vi "WILT Update Wilt GUI.vi"(0 "Dryer In":T1 {"Night Cycle Count" format="%04d"; "Day Cycle Count" format="%04d"}, 1 "Day Shift?":bool, 2 "Enum":T7, 3 "Station Index":i32=13, 5 "Station Label In":string, 7 "New Dryer Details In":T2, 9 "Com Port In":u8=13, 11 "Dryer Status Serial Data In":T5, 12 "Agilent Data In":dbl[](array[numeric])=[1.0, 2.0, 3.0, 4.0, 5.0], 13 "Audit Alert":bool) -> (4 "Dryer Out 2":T1 {"Night Cycle Count" format="%04d"; "Day Cycle Count" format="%04d"}, 8 "New Dryer Testing File Init":bool, 10 "Restart Ready?":bool)   [LabVIEW 2016]
uses:
  Type Definitions/WILT Dryer Status Ctrl.ctl
  Globals/Globals Wilt.vi
  Type Definitions/WILT Dryer.ctl
  Type Definitions/WILT Dryer Details.ctl
  Type Definitions/WILT Dryer Com Port Info.ctl
  Type Definitions/WILT Update GUI Control.ctl
  Type Definitions/WILT Agilent Channel Definition.ctl
  Type Definitions/WILT DAQ Data.ctl
panel:
  in  "Tab Control":enum32{"Out", "In"}(tab)
  out "Dryer Breakout":T1 {"Night Cycle Count" format="%04d"; "Day Cycle Count" format="%04d"}
  in  "Dryer Out":T1 {"Night Cycle Count" format="%04d"; "Day Cycle Count" format="%04d"}
  out "Dryer Breakout":T1 {"Night Cycle Count" format="%04d"; "Day Cycle Count" format="%04d"}
  in  "Dryer":T1 {"Night Cycle Count" format="%04d"; "Day Cycle Count" format="%04d"}
  # "Day"
  # "Night"
  # "Day"
  # "Night"
  # "Day"
  # "Night"
  # "Day"
  # "Night"
  # "Day"
  # "Night"
  # "Day"
  # "Night"
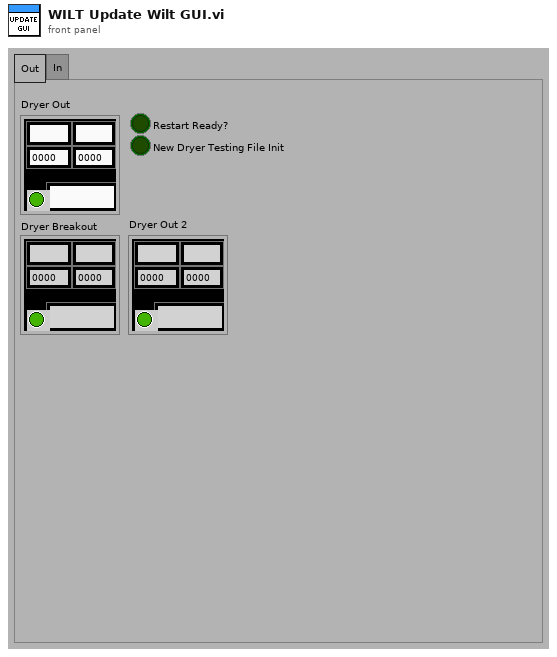
[diagram p1: front panel]
types:
  T1 = typedef "WILT Dryer.ctl" = cluster{"Lab ID":string, "Day Cycle Count":i32, "Station Label":string, "Dryer Details":T2, "Status Color":u32, "Invisible Button":bool, "Night Cycle Count":i32, "Station Index":i32, "Cycle Index":string, "Audit Alert":bool, "Agilent Channel Definition":T3, "DAQ Data":T4}
  T2 = typedef "WILT Dryer Details.ctl" = cluster{"Station":string, "Lab ID":string, "TR Number":string}
  T3 = typedef "WILT Agilent Channel Definition.ctl" = cluster{"Channel":string, "Station":string, "Label":string, "Agilent Station":string, "Data":dbl}
  T4 = typedef "WILT DAQ Data.ctl" = cluster{"L1 Current":dbl, "L2 Current":dbl, "Temperature  Deg F (TC)":dbl, "Volts":dbl, "Volts (208)":dbl, "SW (208)":dbl}
  T5 = typedef "WILT Dryer Com Port Info.ctl" = cluster{"Color":u32, "Last Read Status":T6, "Command:Data":string, "Com Port":u8, "Time(S)":dbl, "Err Count":u32}
  T6 = typedef "WILT Dryer Status Ctrl.ctl" = enum16{"Cycle Not Started", "Cycle Running", "Paused", "Cycle Completed", "Eval Mode Entered", "Err", "Pause (No GEA2)"}
  T7 = typedef "WILT Update GUI Control.ctl" = enum16{"Init Station Number", "Update Detail Data", "Update Status", "Init Com Port Num", "Update Sample Info", "Reset All Cycles"}
  T8 = cluster{"New Dryer Details In":T2, "Station Label In":string, "Com Port In":u8, "Agilent Data In":dbl[], "Dryer Status Serial Data In":T5, "Restart Ready?":bool, "Dryer Out":T1, "Temperature Fault":bool, "Station Index":i32, "Audit Alert":bool, "Day Shift?":bool}
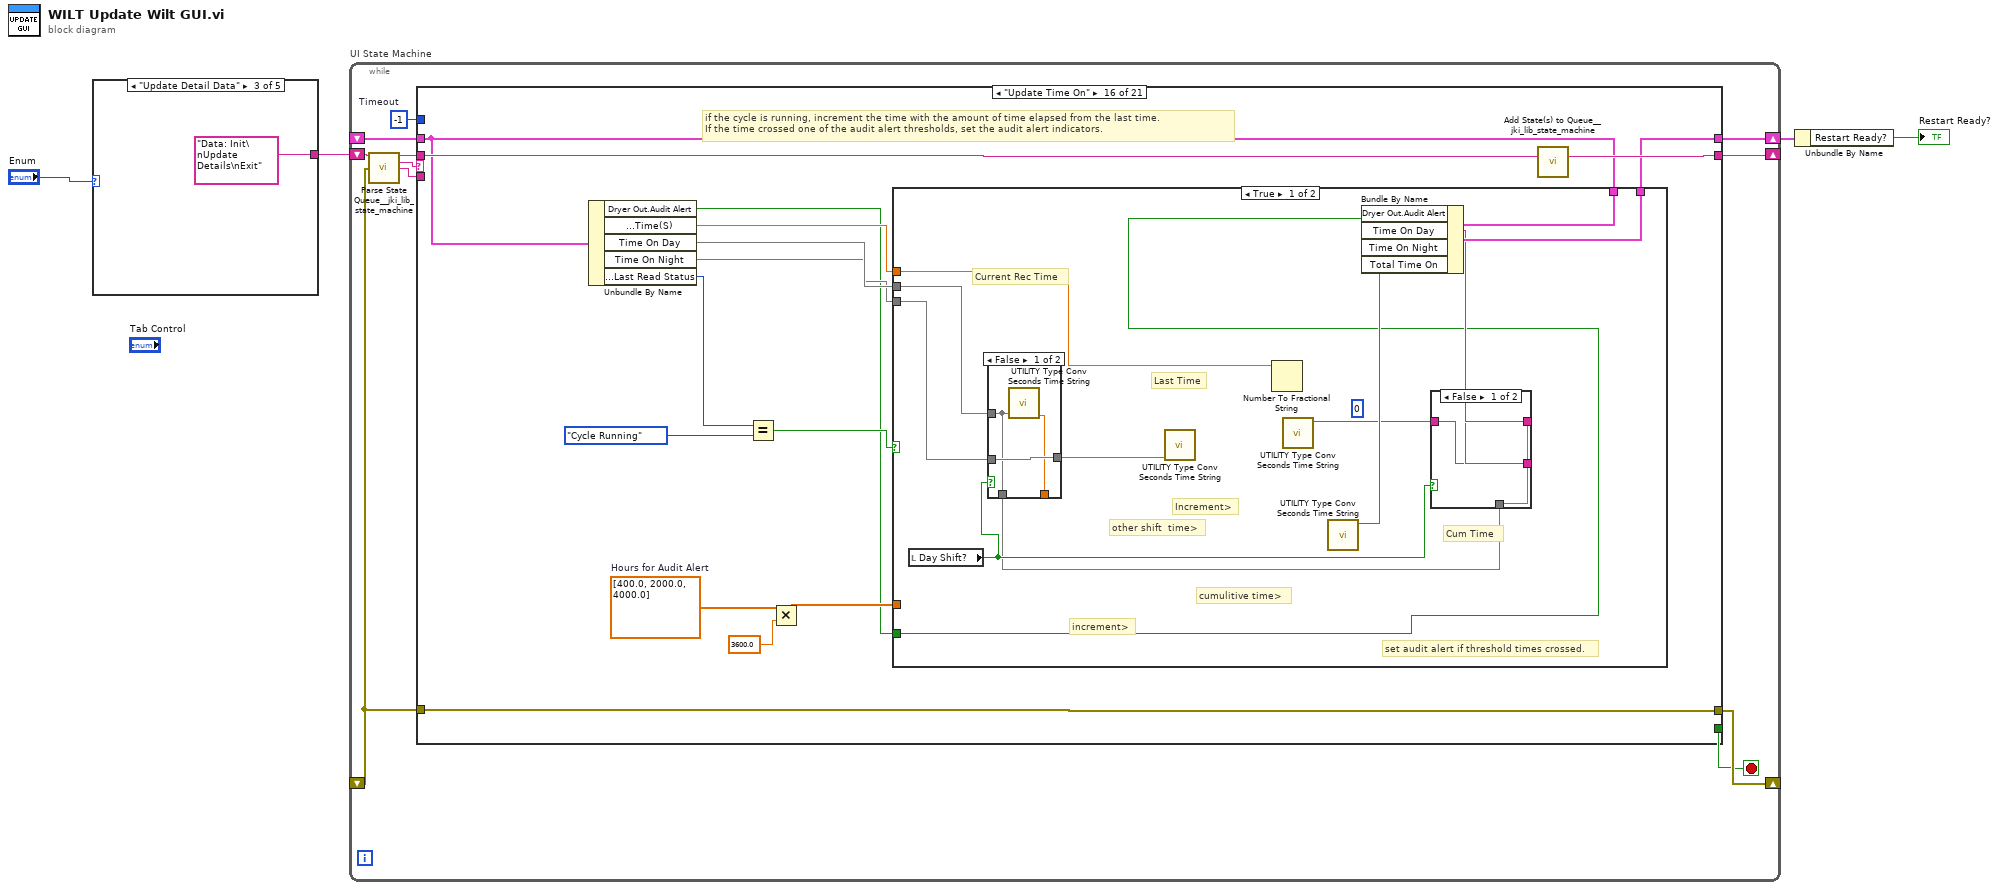
[diagram p0: block diagram]
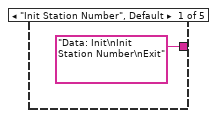
[diagram p2: hidden frame]
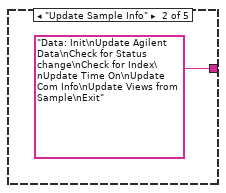
[diagram p3: hidden frame]
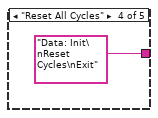
[diagram p4: hidden frame]
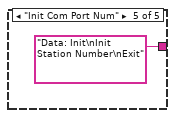
[diagram p5: hidden frame]
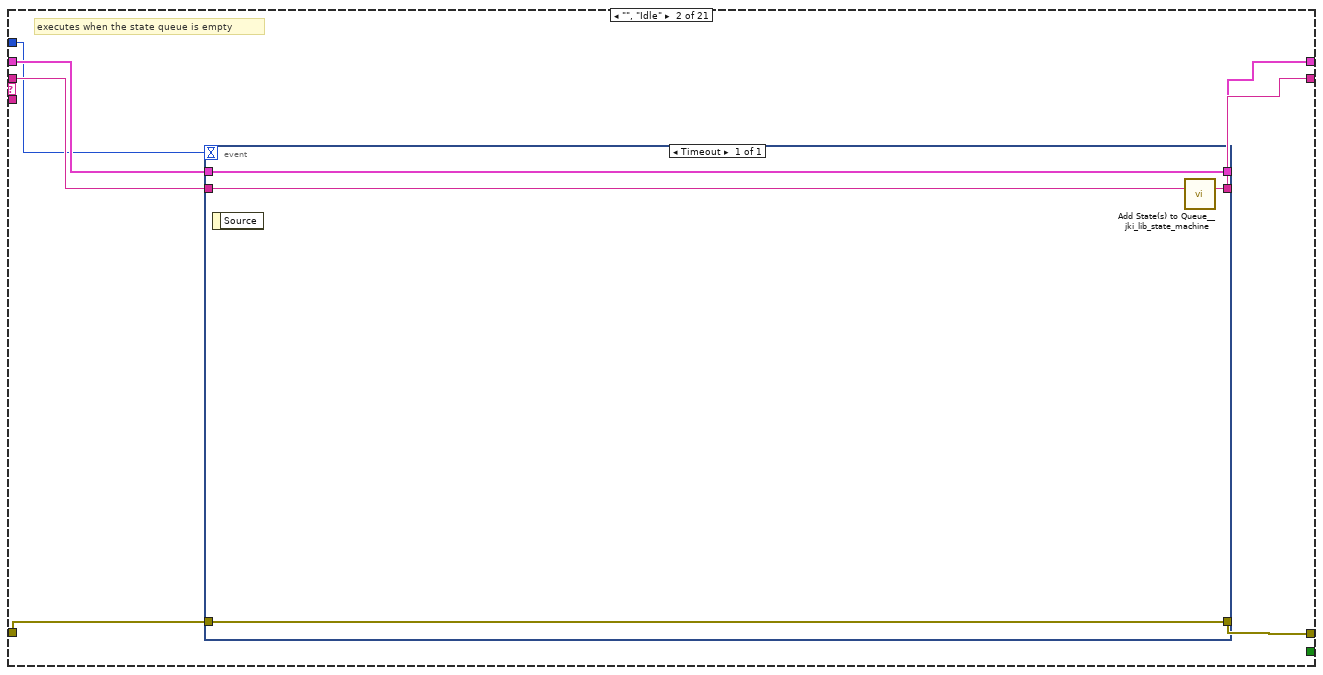
[diagram p7: hidden frame]
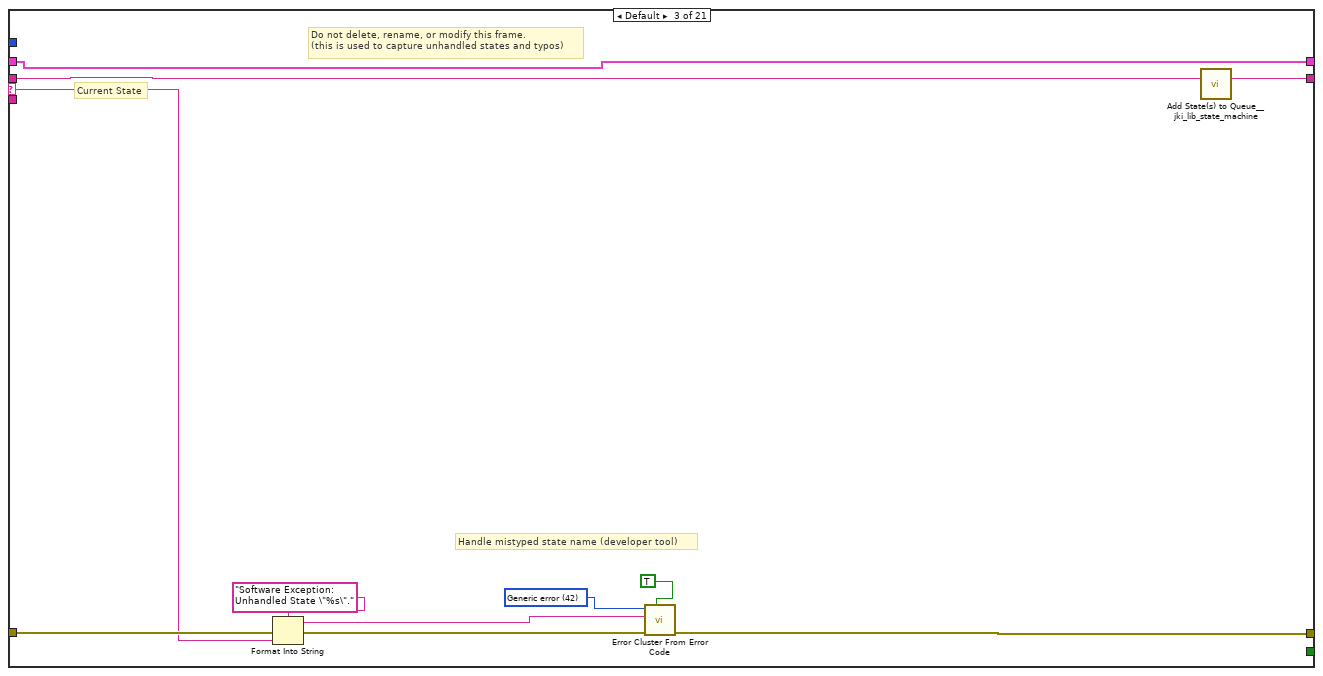
[diagram p8: hidden frame]
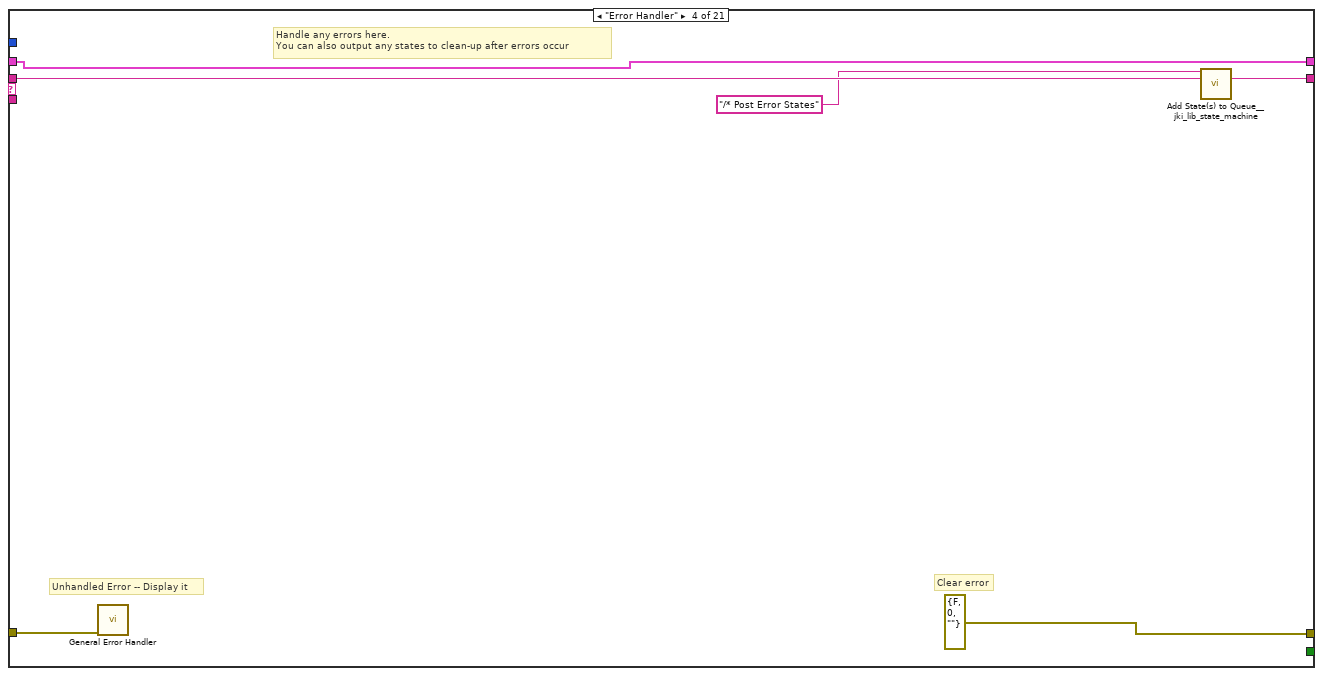
[diagram p9: hidden frame]
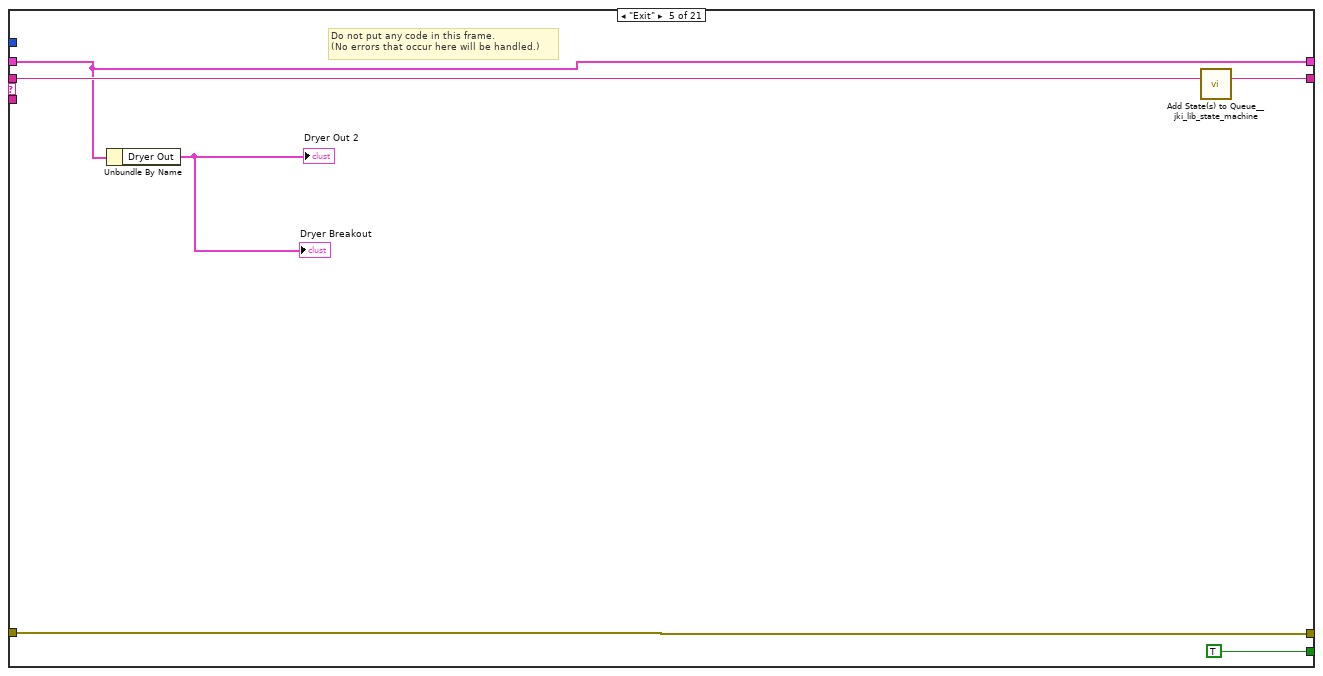
[diagram p10: hidden frame]
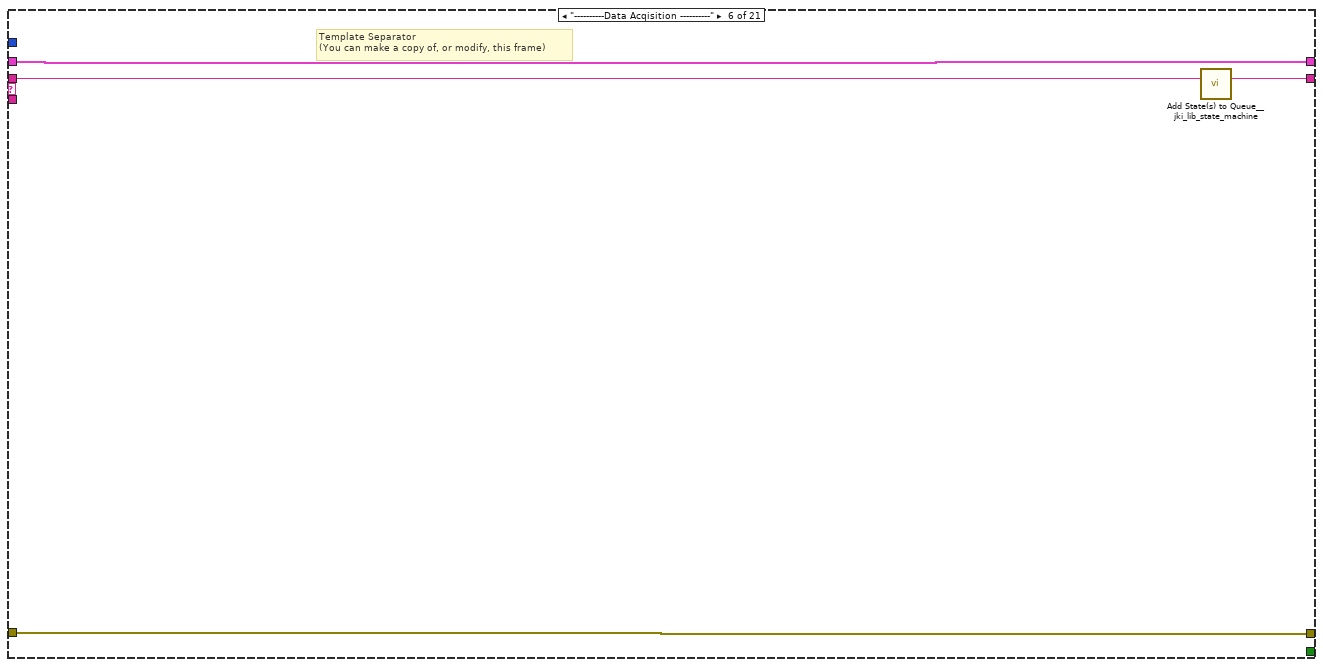
[diagram p11: hidden frame]
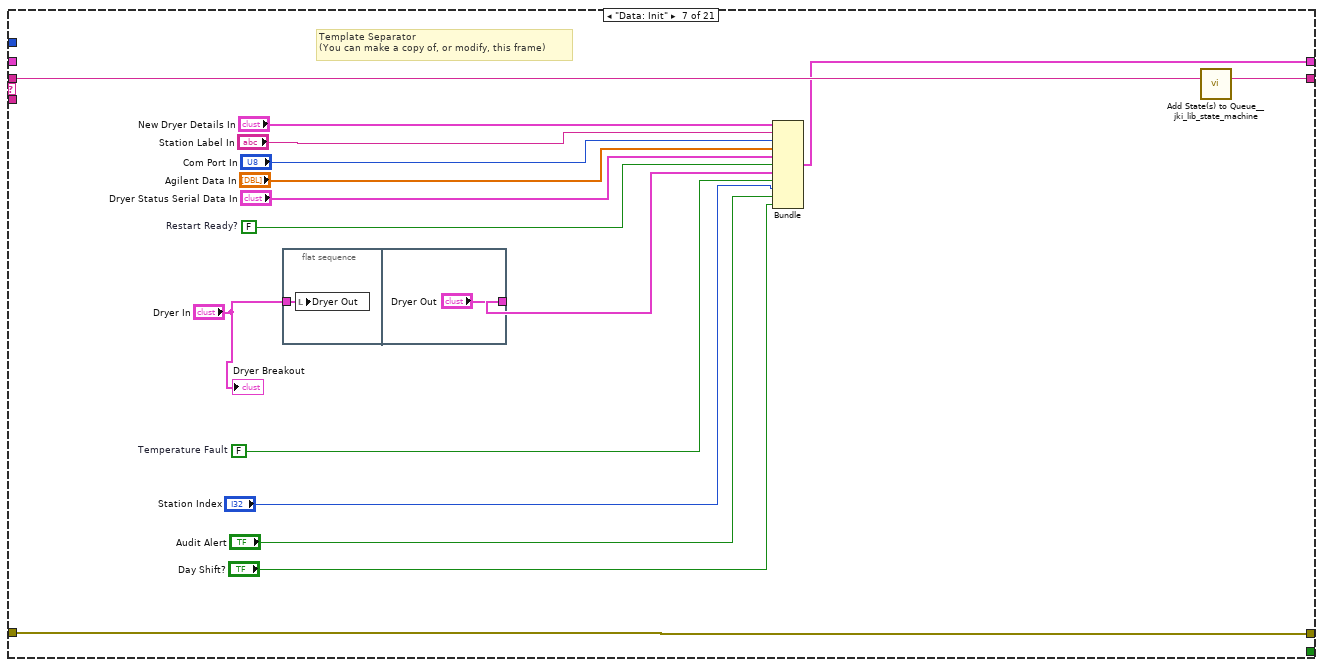
[diagram p12: hidden frame]
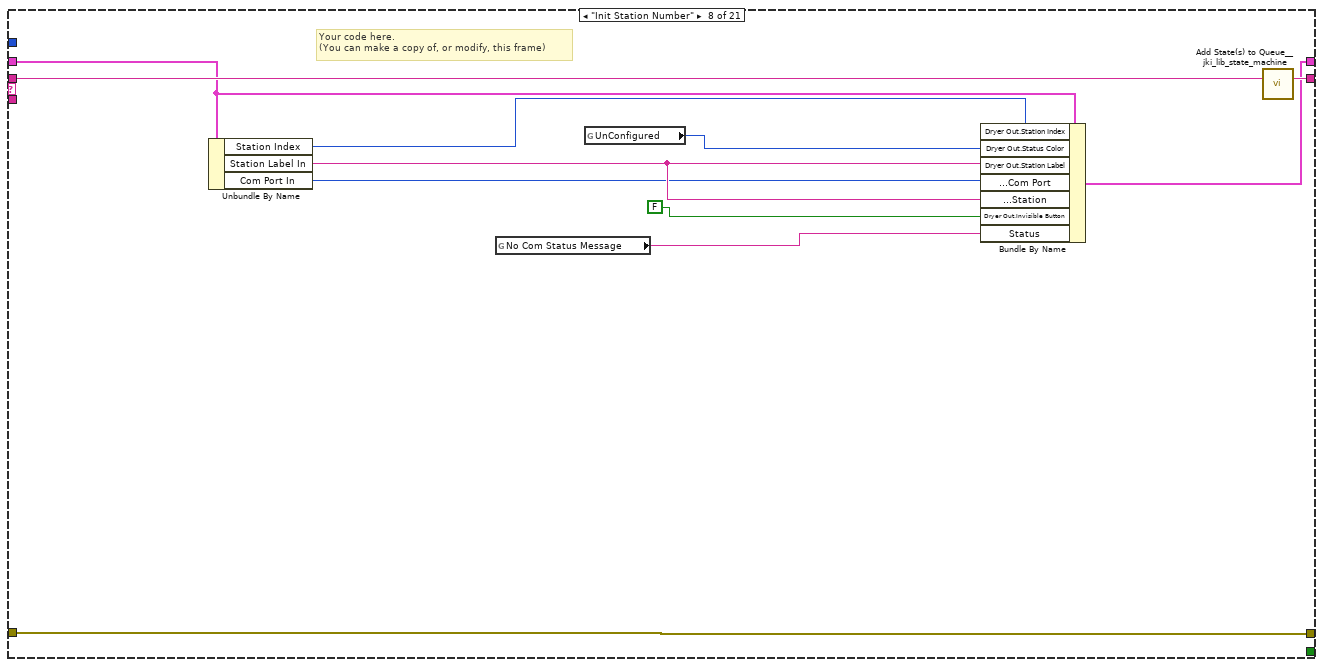
[diagram p13: hidden frame]
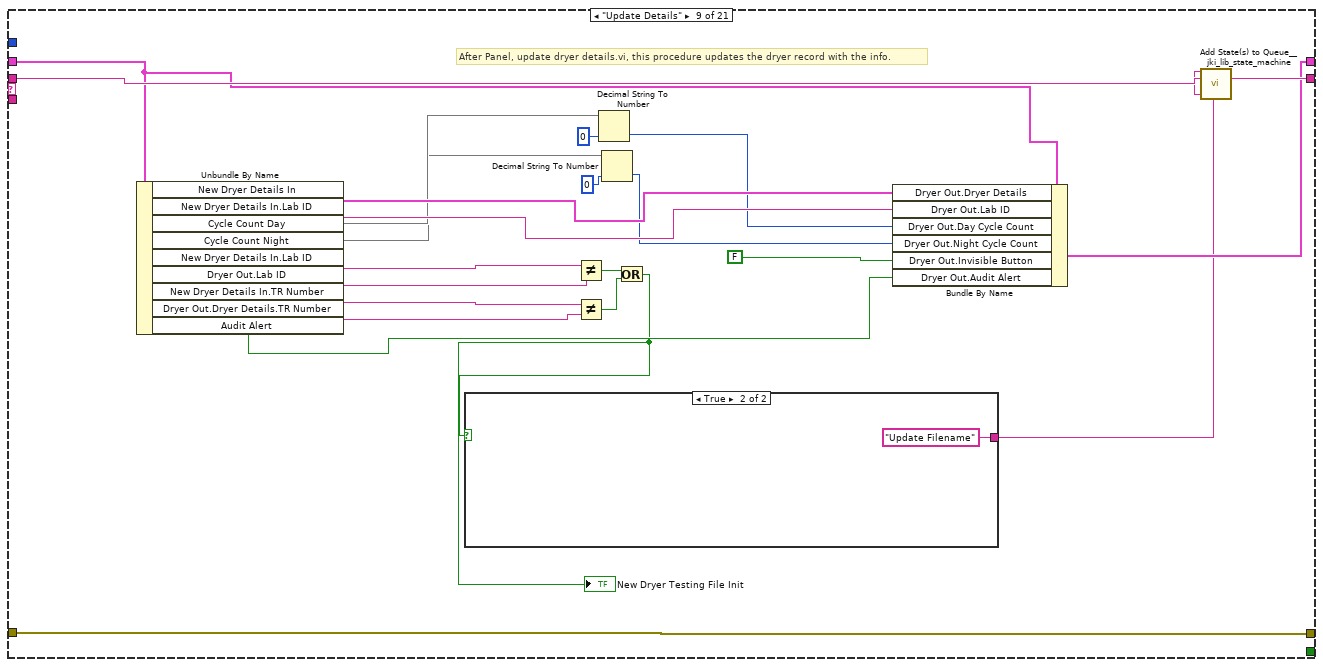
[diagram p14: hidden frame]
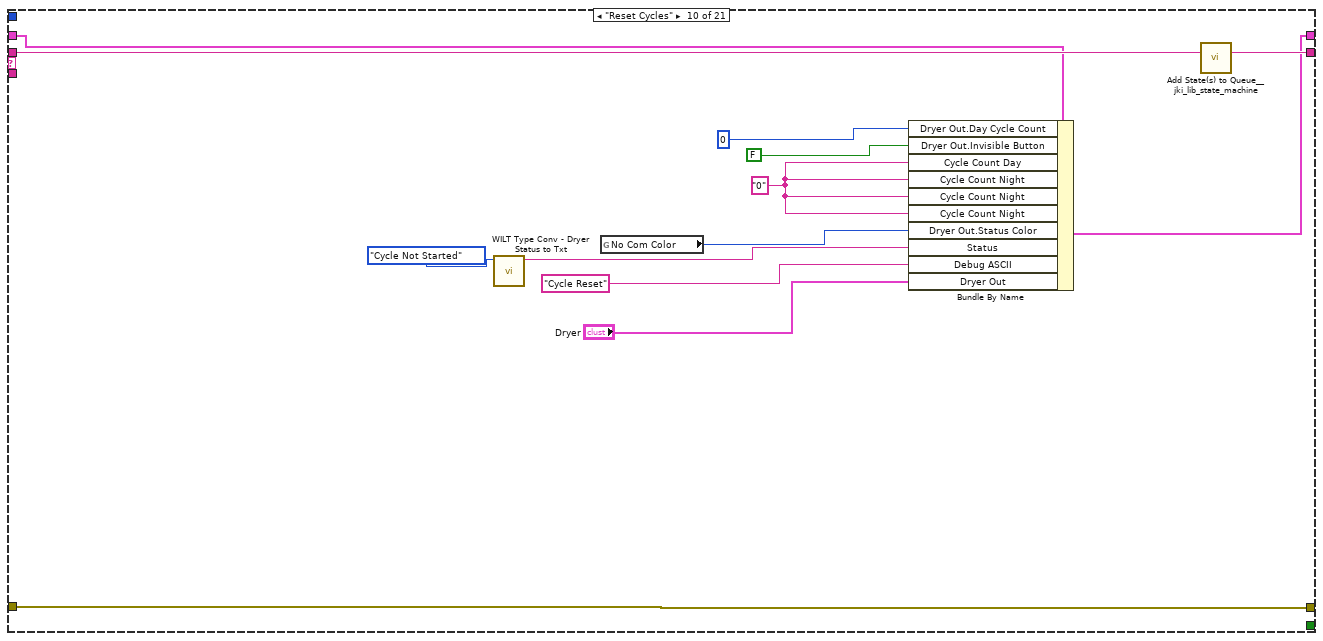
[diagram p16: hidden frame]
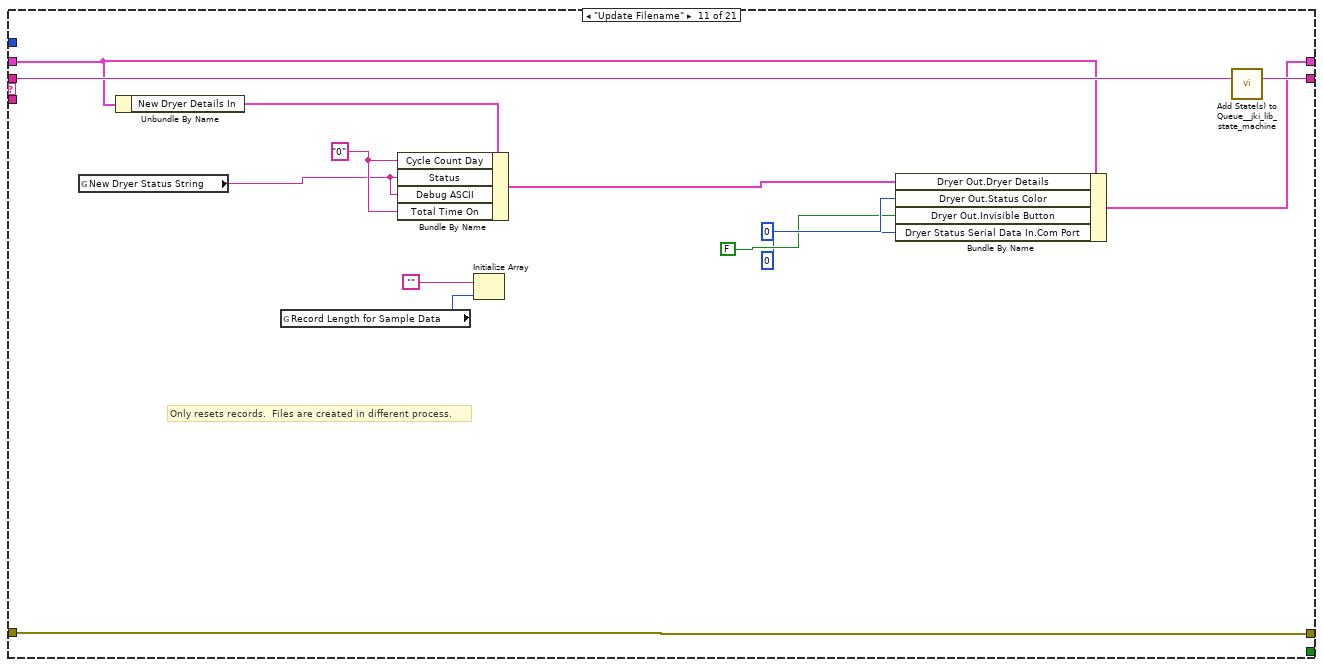
[diagram p17: hidden frame]
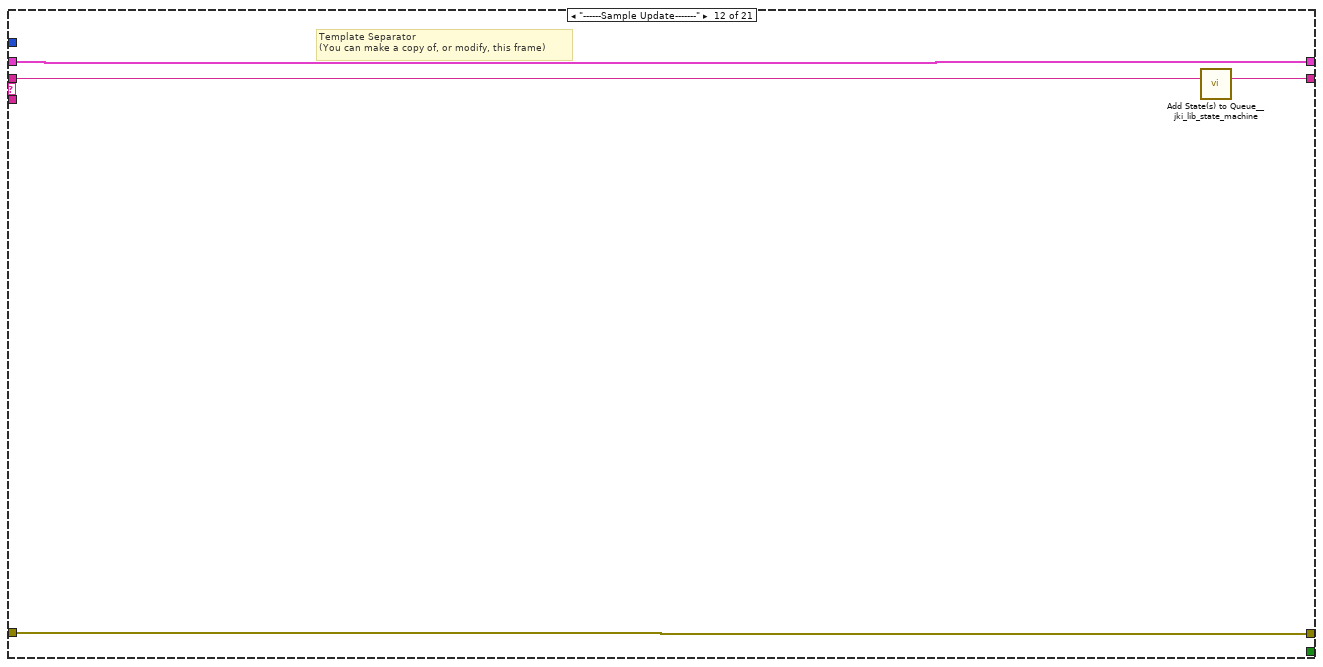
[diagram p18: hidden frame]
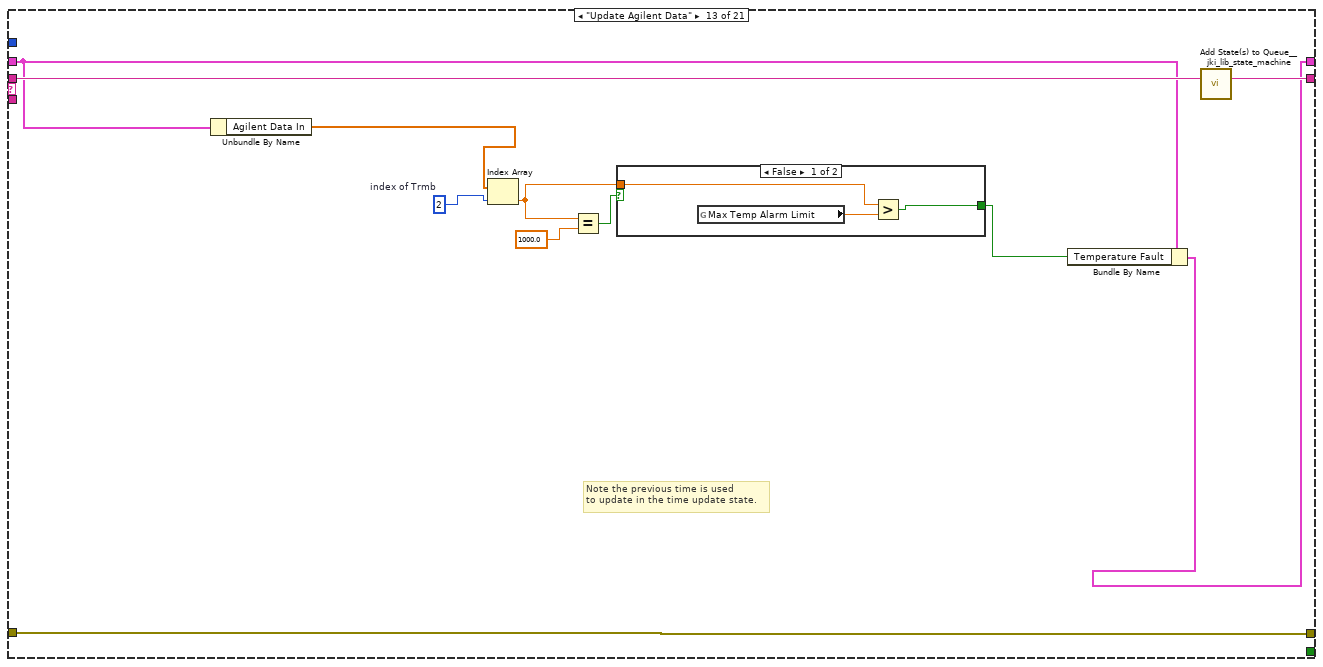
[diagram p19: hidden frame]
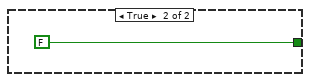
[diagram p20: hidden frame]
diagram:
  n1 = case shown="\"Update Detail Data\"" "Enum" {
    tunnel: ["Data: Init\nInit Station Number\nExit" ("States Out") "Data: Init\nUpdate Agilent Data\nCheck for Status change\nCheck for Index\nUpdate Time On\nUpdate Com Info\nUpdate Views from Sample\nExit" ("States Out") "Data: Init\nUpdate Details\nExit" ("States Out") "Data: Init\nReset Cycles\nExit" ("States Out") "Data: Init\nInit Station Number\nExit" ("States Out")] -> w3
    frame "Init Station Number", Default {
    }
    frame "Update Sample Info" {
    }
    frame "Update Detail Data" {
    }
    frame "Reset All Cycles" {
    }
    frame "Init Com Port Num" {
    }
  }
  n2 = while "UI State Machine" {
    shift-right: [w13] -> w2
    shift-left: _ -> [w12]
    shift-right: [w16] -> _
    shift-left: _ -> [w10]
    shift-right: [w15] -> _
    shift-left: w3 -> [w17]
    stop <- w14 stop-if-true
    w11 = -1  # Timeout
    n3 = call <vilib>:"Parse State Queue__jki_lib_state_machine.vi"("State Queue"=w17, "Error In (no error)"=w10) -> ("Remaining States"=w19:string, "Current State"=w20:string, "Arguments"=w18:string)  [unwired: 11 in]
    n4 = case shown="\"Update Time On\"" w20 {
      selector: w20 -> [_ _ w35 _ _ _ _ _ _ _ _ _ _ _ _ _ _ _ _ _ _]
      tunnel: w19 -> [w22 w30 w39 w51 w57 w61 w77 w90 w113 w127 w141 w145 w156 w164 w168 w183 w223 w227 w231 w238 w254]
      tunnel: w18 -> [_ _ _ _ _ _ _ _ _ _ _ _ _ _ _ _ _ _ _ _ _]
      tunnel: w12 -> [w23 w28 w37 w48 w53 w58 _ w80 w106 w117 w138 w142 w152 w161 w165 w178 w220 w224 w228 w232 w251]
      tunnel: [w21 w27 w41 errorcluster {"status"=FALSE, "code"=0, "source"=""} ("error out") w55 w59 w75 w88 w111 w125 w139 w143 w154 w162 w166 w181 w221 w225 w229 w236 w252] -> w16
      tunnel: w10 -> [w21 w26 w40 w47 w55 w59 w75 w88 w111 w125 w139 w143 w154 w162 w166 w181 w221 w225 w229 w236 w252]
      tunnel: [w22 w29 w38 w50 w56 w60 w76 w89 w112 w126 w140 w144 w155 w163 w167 w182 w222 w226 w230 w237 w253] -> w15
      tunnel: [_ _ _ _ TRUE _ _ _ _ _ _ _ _ _ _ _ _ _ _ _ _] -> w14
      tunnel: [w23 w25 w37 w48 w53 w58 w74 w87 w110 w124 w137 w142 w146 w161 w165 w177 w219 w224 w228 w232 w250] -> w13
      tunnel: w11 -> [_ w24 _ _ _ _ _ _ _ _ _ _ _ _ _ _ _ _ _ _ _]
      frame "ABOUT" {
        # "TAKES DATA FROM DRYER COM INFO AND INTEGRATES IT INTO THE RECORD."
        # "Update Dryer WILT data structure\nwith new data, or init:"
      }
      frame "", "Idle" {
        # "executes when the state queue is empty"
        n5 = event shown="[0] Timeout" {
          selector: _ -> [_]
          dyn-events: _ -> [_]
          timeout: w24 -> [_]
          tunnel: w30 -> [w34]
          tunnel: [w33] -> w29
          tunnel: w28 -> [w31]
          tunnel: [w32] -> w27
          tunnel: w26 -> [w32]
          tunnel: [w31] -> w25
          event Timeout {
            n6 = event-data() -> ()  [unwired: 1 in, 1 out]
            n7 = call <vilib>:"Add State(s) to Queue__jki_lib_state_machine.vi"("State(s) in (\"\")"=w34) -> ("States Out"=w33:string)  [unwired: 14 in]
          }
        }
      }
      frame Default {
        w44 = 42 items=["No error", "Argument error", "Memory is full", "Out of zone", "End of file", "File already open", "Generic file I/O error", "File not found", "File permission error", "Disk is full", "Duplicate path", "Too many files open", "System feature not enabled", "Resource file not found", "Cannot add resource", "Resource not found", "Image not found", "Image memory error", "Pen does not exist", "Config type invalid", "Config token not found", "Config parse error", "Config memory error", "Bad external code format", "Bad external code offset", "External code not present", "Null window", "Destroy window error", "Null menu", "Print aborted", "Bad print record", "Print driver error", "Windows error during printing", "Memory error during printing", "Print dialog error", "Generic print error", "Invalid device refnum", "Device not found", "Device parameter error", "Device unit error", "Cannot open device", "Device call aborted", "Generic error", "Cancelled by user", "Object ID too low", "Object ID too high", "Object not in heap", "Unknown heap", "Unknown object (invalid DefProc)", "Unknown object (DefProc not in table)", "Message out of range", "Invalid (null) method", "Unknown message", "Manager call not supported", "Bad address", "Network operation in progress", "Network operation timed out", "Connection is busy", "Network attribute not supported", "Network error", "Address in use", "System out of memory", "Connection aborted", "Connection refused", "Not connected", "Already connected", "Connection closed", "Initialization error (interapplication manager)", "Bad occurrence", "Wait on unbound occurrence handler", "Occurrence queue overflow", "Datalog type conflict", "Unused", "Unrecognized type (interapplication manager)", "Memory corrupt", "Failed to make temporary DLL", "Old CIN version", "Drag socket not found", "Failed to load drop-object", "Failed to register OLE object", "Failed to release OLE object", "Format specifier type mismatch", "Unknown format specifier", "Too few format specifiers", "Too many format specifiers", "Scan failed", "Newer CIN version", "Error converting to variant", "Runtime menu error", "Password tampered", "Variant attribute not found", "Incompatible variant data type", "Event data is not available", "Event Store is not present", "Occurrence is not found", "Event Queue is not created", "Event info is not available", "Refnum passed is NULL", "Error retrieving Class GUID", "Error retrieving CoClass GUID", "Error retrieving TypeLib GUID.", "Bad built application magic bytes.", "Specific driver is different from the specific driver associated with the Logical Name.", "There is no session opened to the class driver.", "Max Error", "MAX - Error with config objects", "MAX - Error loading configuration", "MAX - Group not supported"]
        # "Current State"
        # "Do not delete, rename, or modify this frame.\n(this is used to capture unhandled states and typos)"
        # "Handle mistyped state name (developer tool)"
        n8 = Format Into String(format string="Software Exception: Unhandled State \"%s\"." ("message"), error in=w40, w35) -> (resulting string=w43:string, error out=w42:errorcluster)  [unwired: 1 in]
        n9 = call <vilib>:"Error Cluster From Error Code.vi"("show call chain? (False)"=TRUE, "error in (no error)"=w42, "error message (\"\")"=w43, "error code (0)"=w44) -> ("error out"=w41:errorcluster)  [unwired: 5 in]
        n10 = call <vilib>:"Add State(s) to Queue__jki_lib_state_machine.vi"("State(s) in (\"\")"=w39) -> ("States Out"=w38:string)  [unwired: 14 in]
      }
      frame "Error Handler" {
        # "Unhandled Error -- Display it"
        # "Handle any errors here.\nYou can also output any states to clean-up after errors occur"
        # "Clear error"
        n11 = call <vilib>:"General Error Handler.vi"("error in (no error)"=w47) -> ()  [unwired: 10 in, 5 out]
        n12 = call <vilib>:"Add State(s) to Queue__jki_lib_state_machine.vi"("State(s) in Front (\"\")"="/* Post Error States", "State(s) in (\"\")"=w51) -> ("States Out"=w50:string)  [unwired: 13 in]
      }
      frame "Exit" {
        # "Do not put any code in this frame.\n(No errors that occur here will be handled.)"
        n13 = Unbundle By Name(w53) -> ("Dryer Out"=→"Dryer Out 2" →"Dryer Breakout":T1)
        n14 = call <vilib>:"Add State(s) to Queue__jki_lib_state_machine.vi"("State(s) in (\"\")"=w57) -> ("States Out"=w56:string)  [unwired: 14 in]
      }
      frame "----------Data Acqisition ----------" {
        # "Template Separator\n(You can make a copy of, or modify, this frame)"
        n15 = call <vilib>:"Add State(s) to Queue__jki_lib_state_machine.vi"("State(s) in (\"\")"=w61) -> ("States Out"=w60:string)  [unwired: 14 in]
      }
      frame "Data: Init" {
        w66 = FALSE  # Temperature Fault
        w69 = FALSE  # Restart Ready?
        # "Template Separator\n(You can make a copy of, or modify, this frame)"
        n16 = flat-sequence {
          tunnel: "Dryer In" -> [w78]
          tunnel: ["Dryer Out"] -> w67
          frame #0 {
            n17 = local write "Dryer Out"(w78) -> ()
          }
          frame #1 {
          }
        }
        n18 = Bundle("New Dryer Details In"="New Dryer Details In", "Station Label In"="Station Label In", "Com Port In"="Com Port In", "Agilent Data In"="Agilent Data In", "Dryer Status Serial Data In"="Dryer Status Serial Data In", "Restart Ready?"=w69, "Dryer Out"=w67, "Temperature Fault"=w66, "Station Index"="Station Index", "Audit Alert"="Audit Alert", "Day Shift?"="Day Shift?") -> (w74:T8)  [unwired: 1 in]
        n19 = call <vilib>:"Add State(s) to Queue__jki_lib_state_machine.vi"("State(s) in (\"\")"=w77) -> ("States Out"=w76:string)  [unwired: 14 in]
        "Dryer Breakout" <- "Dryer In"
      }
      frame "Init Station Number" {
        # "Your code here.\n(You can make a copy of, or modify, this frame)"
        n20 = Unbundle By Name(w80) -> ("Station Index"=w81:i32, "Station Label In"=w83:string, "Com Port In"=w82:u8)
        n21 = global read "Globals Wilt.vi" "No Com Status Message"() -> (w84:string)
        n22 = global read "Globals Wilt.vi" "UnConfigured"() -> (w85:u32)
        n23 = Bundle By Name(cluster=w80, "Dryer Out.Station Index"=w81, "Dryer Out.Status Color"=w85, "Dryer Out.Station Label"=w83, "Dryer Status Serial Data In.Com Port"=w82, "Dryer Out.Dryer Details.Station"=w83, "Dryer Out.Invisible Button"=FALSE ("Dryer In.Boolean"), "Status"=w84) -> (w87:T8)
        n24 = call <vilib>:"Add State(s) to Queue__jki_lib_state_machine.vi"("State(s) in (\"\")"=w90) -> ("States Out"=w89:string)  [unwired: 14 in]
      }
      frame "Update Details" {
        # "After Panel, update dryer details.vi, this procedure updates the dryer record with the info."
        n25 = Unbundle By Name(w106) -> ("New Dryer Details In"=w102:T2, "New Dryer Details In.Lab ID"=w100:string, "Cycle Count Day"=w99, "Cycle Count Night"=w96, "New Dryer Details In.Lab ID"=w94:string, "Dryer Out.Lab ID"=w93:string, "New Dryer Details In.TR Number"=w95:string, "Dryer Out.Dryer Details.TR Number"=w105:string, "Audit Alert"=w92:bool)
        n26 = Not Equal?(x=w94, y=w93) -> (x != y?=w104:bool)
        n27 = Not Equal?(x=w95, y=w105) -> (x != y?=w103:bool)
        n28 = Decimal String To Number(string=w99, default (0L)=0 ("default (0 I32)")) -> (number=w98:i32)  [unwired: 1 in, 1 out]
        n29 = Decimal String To Number(string=w96, default (0L)=0 ("default (0 I32)")) -> (number=w97:i32)  [unwired: 1 in, 1 out]
        n30 = Or(x=w104, y=w103) -> (x .or. y?=w91:bool)
        "New Dryer Testing File Init" <- w91
        n31 = case shown="True" w91 {
          tunnel: [_ "Update Filename"] -> w109
          frame False {
          }
          frame True {
          }
        }
        n32 = Bundle By Name(cluster=w106, "Dryer Out.Dryer Details"=w102, "Dryer Out.Lab ID"=w100, "Dryer Out.Day Cycle Count"=w98, "Dryer Out.Night Cycle Count"=w97, "Dryer Out.Invisible Button"=FALSE ("Dryer In.Boolean"), "Dryer Out.Audit Alert"=w92) -> (w110:T8)
        n33 = call <vilib>:"Add State(s) to Queue__jki_lib_state_machine.vi"("State(s) in Front (\"\")"=w109, "State(s) in (\"\")"=w113) -> ("States Out"=w112:string)  [unwired: 13 in]
      }
      frame "Reset Cycles" {
        w115 = "0" ("Dryer Out.Dryer Details.Cycle Count")
        n34 = call "WILT Type Conv - Dryer Status to Txt.vi"("Status"=WILT_Dryer_Status_Ctrl."Cycle Not Started") -> ("Ring Text.Text"=w119:string)  [unwired: 10 in]
        n35 = global read "Globals Wilt.vi" "No Com Color"() -> (w121:u32)
        n36 = Bundle By Name(cluster=w117, "Dryer Out.Day Cycle Count"=0 ("Dryer Out.Cycle Count"), "Dryer Out.Invisible Button"=FALSE ("Dryer In.Boolean"), "Cycle Count Day"=w115, "Cycle Count Night"=w115, "Cycle Count Night"=w115, "Cycle Count Night"=w115, "Dryer Out.Status Color"=w121, "Status"=w119, "Debug ASCII"="Cycle Reset" ("Dryer Out.Dryer Details.Debug ASCII"), "Dryer Out"="Dryer") -> (w124:T8)
        n37 = call <vilib>:"Add State(s) to Queue__jki_lib_state_machine.vi"("State(s) in (\"\")"=w127) -> ("States Out"=w126:string)  [unwired: 14 in]
      }
      frame "Update Filename" {
        w136 = "0" ("Cycle Count")
        # "Only resets records.  Files are created in different process."
        n38 = global read "Globals Wilt.vi" "New Dryer Status String"() -> (w128:string)
        n39 = Unbundle By Name(w138) -> ("New Dryer Details In"=w134:T2)
        n40 = global read "Globals Wilt.vi" "Record Length for Sample Data"() -> (w129:i32)
        n41 = Bundle By Name(cluster=w134, "Cycle Count Day"=w136, "Status"=w128, "Debug ASCII"=w128, "Total Time On"=w136) -> (w135:T2)
        n42 = Initialize Array("", w129) -> ()  [unwired: 1 out]
        n43 = Bundle By Name(cluster=w138, "Dryer Out.Dryer Details"=w135, "Dryer Out.Status Color"=u32 0 ("Dryer In.Status Color"), "Dryer Out.Invisible Button"=FALSE ("Dryer In.Boolean"), "Dryer Status Serial Data In.Com Port"=u8 0 ("Dryer In.Com Port")) -> (w137:T8)
        n44 = call <vilib>:"Add State(s) to Queue__jki_lib_state_machine.vi"("State(s) in (\"\")"=w141) -> ("States Out"=w140:string)  [unwired: 14 in]
      }
      frame "------Sample Update-------" {
        # "Template Separator\n(You can make a copy of, or modify, this frame)"
        n45 = call <vilib>:"Add State(s) to Queue__jki_lib_state_machine.vi"("State(s) in (\"\")"=w145) -> ("States Out"=w144:string)  [unwired: 14 in]
      }
      frame "Update Agilent Data" {
        w151 = 2  # index of Trmb
        # "Note the previous time is used\nto update in the time update state."
        n46 = Unbundle By Name(w152) -> ("Agilent Data In"=w153:dbl[])
        n47 = Index Array(array=w153, index=w151) -> (element=w147:dbl)
        n48 = Equal?(x=w147, y=1000.0) -> (x = y?=w149:bool)
        n49 = case shown="False" w149 {
          tunnel: [w157 FALSE] -> w148
          tunnel: w147 -> [w158 _]
          frame False {
            n50 = global read "Globals Wilt.vi" "Max Temp Alarm Limit"() -> (w159:dbl)
            n51 = Greater?(x=w158, y=w159) -> (0:w157:bool)
          }
          frame True {
          }
        }
        n52 = Bundle By Name(cluster=w152, "Temperature Fault"=w148) -> (w146:T8)
        n53 = call <vilib>:"Add State(s) to Queue__jki_lib_state_machine.vi"("State(s) in (\"\")"=w156) -> ("States Out"=w155:string)  [unwired: 14 in]
      }
      frame "Check for Status change" {
        # "If the status string changes from:\n1. running to complete: set restart ready\n2. complete to running: go to increment count."
        n54 = Unbundle By Name(w161) -> ()  [unwired: 1 out]
        n55 = call <vilib>:"Add State(s) to Queue__jki_lib_state_machine.vi"("State(s) in (\"\")"=w164) -> ("States Out"=w163:string)  [unwired: 14 in]
      }
      frame "Check for Index" {
        # "Your code here.\n(You can make a copy of, or modify, this frame)"
        n56 = call <vilib>:"Add State(s) to Queue__jki_lib_state_machine.vi"("State(s) in (\"\")"=w168) -> ("States Out"=w167:string)  [unwired: 14 in]
      }
      frame "Update Time On" {
        w172 = dbl[] [400.0, 2000.0, 4000.0]  # Hours for Audit Alert
        # "if the cycle is running, increment the time with the amount of time elapsed from the last time. \nIf the time crossed one of the audit alert thresholds, set the audit alert indicators."
        n57 = Unbundle By Name(w178) -> ("Dryer Out.Audit Alert"=w169:bool, "Dryer Status Serial Data In.Time(S)"=w179:dbl, "Time On Day"=w174, "Time On Night"=w173, "Dryer Status Serial Data In.Last Read Status"=w175:T6)
        n58 = Equal?(x=w175, y=WILT_Dryer_Status_Ctrl."Cycle Running" ("Status")) -> (x = y?=w180:bool)
        n59 = Multiply(x=w172, y=3600.0 ("Seconds Out")) -> (x*y=w170:dbl[])
        n60 = case shown="True" w180 {
          tunnel: w179 -> [w194 _]
          tunnel: w178 -> [w196 w207]
          tunnel: [w195 w207] -> w177
          tunnel: w174 -> [w193 _]
          tunnel: w173 -> [w191 _]
          tunnel: w170 -> [_ _]
          tunnel: w169 -> [w184 _]
          frame True {
            (unwired) 0 ("index")
            # "increment>"
            # "cumulitive time>"
            # "set audit alert if threshold times crossed."
            # "Increment>"
            # "other shift  time>"
            # "Cum Time"
            # "Current Rec Time"
            # "Last Time"
            n61 = local read "Day Shift?"() -> (w190:bool)
            n62 = case shown="False" w190 {
              tunnel: w193 -> [w201 w206]
              tunnel: [w203 w206] -> w192
              tunnel: w191 -> [w203 w204]
              tunnel: [w202 w205] -> _
              tunnel: [w201 w204] -> w185
              frame False {
                n63 = call "UTILITY Type Conv Seconds Time String.vi"("Time String In"=w201) -> ("Seconds Out"=w202:dbl)  [unwired: 9 in, 1 out]
              }
              frame True {
                n64 = call "UTILITY Type Conv Seconds Time String.vi"("Time String In"=w204) -> ("Seconds Out"=w205:dbl)  [unwired: 9 in, 1 out]
              }
            }
            n65 = call "UTILITY Type Conv Seconds Time String.vi"("Time String In"=w192) -> ()  [unwired: 9 in, 2 out]
            n66 = Number To Fractional String(number=w194) -> ()  [unwired: 3 in, 1 out]
            n67 = call "UTILITY Type Conv Seconds Time String.vi"() -> ("Time String Out"=w187:string)  [unwired: 10 in, 1 out]
            n68 = call "UTILITY Type Conv Seconds Time String.vi"() -> ("Time String Out"=w189:string)  [unwired: 10 in, 1 out]
            n69 = case shown="False" w190 {
              tunnel: [w197 w200] -> w188
              tunnel: w187 -> [w198 w200]
              tunnel: [w198 w199] -> w186
              tunnel: w185 -> [w197 w199]
              frame False {
              }
              frame True {
              }
            }
            n70 = Bundle By Name(cluster=w196, "Dryer Out.Audit Alert"=w184, "Time On Day"=w188, "Time On Night"=w186, "Total Time On"=w189) -> (w195:T8)
          }
          frame False {
          }
        }
        n71 = call <vilib>:"Add State(s) to Queue__jki_lib_state_machine.vi"("State(s) in (\"\")"=w183) -> ("States Out"=w182:string)  [unwired: 14 in]
      }
      frame "Update Com Info" {
        w208 = " :: " ("replace string (\"\")")
        # "Put Dryer Serial Data in into dryer out sample record."
        # "Your code here.\n(You can make a copy of, or modify, this frame)"
        n72 = Unbundle By Name(w220) -> ("Temperature Fault"=w214:bool, "Dryer Status Serial Data In"=w218:T5)
        n73 = Unbundle By Name(w218) -> ("Err Count"=w217:u32, "Color"=w215:u32, "Command:Data"=w216:string)  [unwired: 1 out]
        n74 = global read "Globals Wilt.vi" "Temperature Fault"() -> (w213:u32)
        n75 = Search and Replace String(input string=w216, search string="\r\n", replace string=w208) -> (result string=w210:string)  [unwired: 5 in, 3 out]
        n76 = Select(t=w213, s=w214, f=w215) -> (s? t:f=w212:u32)
        n77 = To Long Integer(number=w217) -> ()  [unwired: 1 out]
        n78 = Search and Replace String(input string=w210, search string="\r", replace string=w208) -> ()  [unwired: 5 in, 4 out]
        n79 = Bundle By Name(cluster=w220, "Dryer Out.Status Color"=w212) -> (w219:T8)
        n80 = call <vilib>:"Add State(s) to Queue__jki_lib_state_machine.vi"("State(s) in (\"\")"=w223) -> ("States Out"=w222:string)  [unwired: 14 in]
      }
      frame "Update Views from Sample" {
        # "Using Sample Record:  Update Dryer Out Record and compare to previous Hist Record to see if max's are exceeded."
        n81 = call <vilib>:"Add State(s) to Queue__jki_lib_state_machine.vi"("State(s) in (\"\")"=w227) -> ("States Out"=w226:string)  [unwired: 14 in]
      }
      frame "-----If Status Has Changed-----" {
        # "Template Separator\n(You can make a copy of, or modify, this frame)"
        n82 = call <vilib>:"Add State(s) to Queue__jki_lib_state_machine.vi"("State(s) in (\"\")"=w231) -> ("States Out"=w230:string)  [unwired: 14 in]
      }
      frame "Update History Data" {
        w233 = "0" ("element")
        # "This may be the memory leak.  Limit the number of  historical records to max record size."
        # "Insert new record on top of stack.  This will be updated as time goes on during the cycle.  This happens when there is an increment count."
        n83 = Unbundle By Name(w232) -> ("Dryer Out.Day Cycle Count"=w234:i32)
        n84 = Number To Fractional String(number=w234) -> (F-format string=w235:string)  [unwired: 3 in]
        n85 = Build Array(w235, w233, w233, w233, w233) -> ()  [unwired: 1 out]
        n86 = call <vilib>:"Add State(s) to Queue__jki_lib_state_machine.vi"("State(s) in (\"\")"=w238) -> ("States Out"=w237:string)  [unwired: 14 in]
      }
      frame "Increment Count" {
        # "Adds one to count in the sample record, and calls update history data (which creates a new history record)."
        n87 = Unbundle By Name(w251) -> ("Cycle Count Day"=w248, "Cycle Count Night"=w247, "Day Shift?"=w239:bool)
        n88 = Decimal String To Number(string=w248) -> (number=w246:i32)  [unwired: 2 in, 1 out]
        n89 = Decimal String To Number(string=w247) -> (number=w245:i32)  [unwired: 2 in, 1 out]
        n90 = case shown="True" w239 {
          tunnel: w246 -> [w255 w260]
          tunnel: w245 -> [w257 w258]
          tunnel: [w255 w259] -> w241
          tunnel: [w256 w258] -> w240
          frame False {
            n91 = Increment(x=w257) -> (x+1=w256:i32)
          }
          frame True {
            n92 = Increment(x=w260) -> (x+1=w259:i32)
          }
        }
        n93 = Add(x=w241, y=w240) -> (x+y=w244:i32)
        n94 = Number To Decimal String(number=w240) -> (decimal integer string=w242:string)  [unwired: 1 in]
        n95 = Number To Decimal String(number=w244) -> ()  [unwired: 1 in, 1 out]
        n96 = Number To Decimal String(number=w241) -> (decimal integer string=w243:string)  [unwired: 1 in]
        n97 = Bundle By Name(cluster=w251, "Cycle Count Day"=w243, "Cycle Count Night"=w242, "Dryer Out.Day Cycle Count"=w241, "Dryer Out.Night Cycle Count"=w240) -> (w250:T8)
        n98 = call <vilib>:"Add State(s) to Queue__jki_lib_state_machine.vi"("State(s) in Front (\"\")"="Update History Data" ("State(s) in Front (\"\")"), "State(s) in (\"\")"=w254) -> ("States Out"=w253:string)  [unwired: 13 in]
      }
    }
  }
  n99 = Unbundle By Name(w2) -> ("Restart Ready?"=→"Restart Ready?":bool)
